vi "Day 03 (Part One).vi"() -> ()   [LabVIEW 2021]
panel:
  out "result":i32
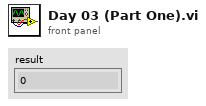
[diagram p1: front panel]
types:
  T1 = cluster{"number":i32, "start index":i32, "lenght":i32, "row":i32}
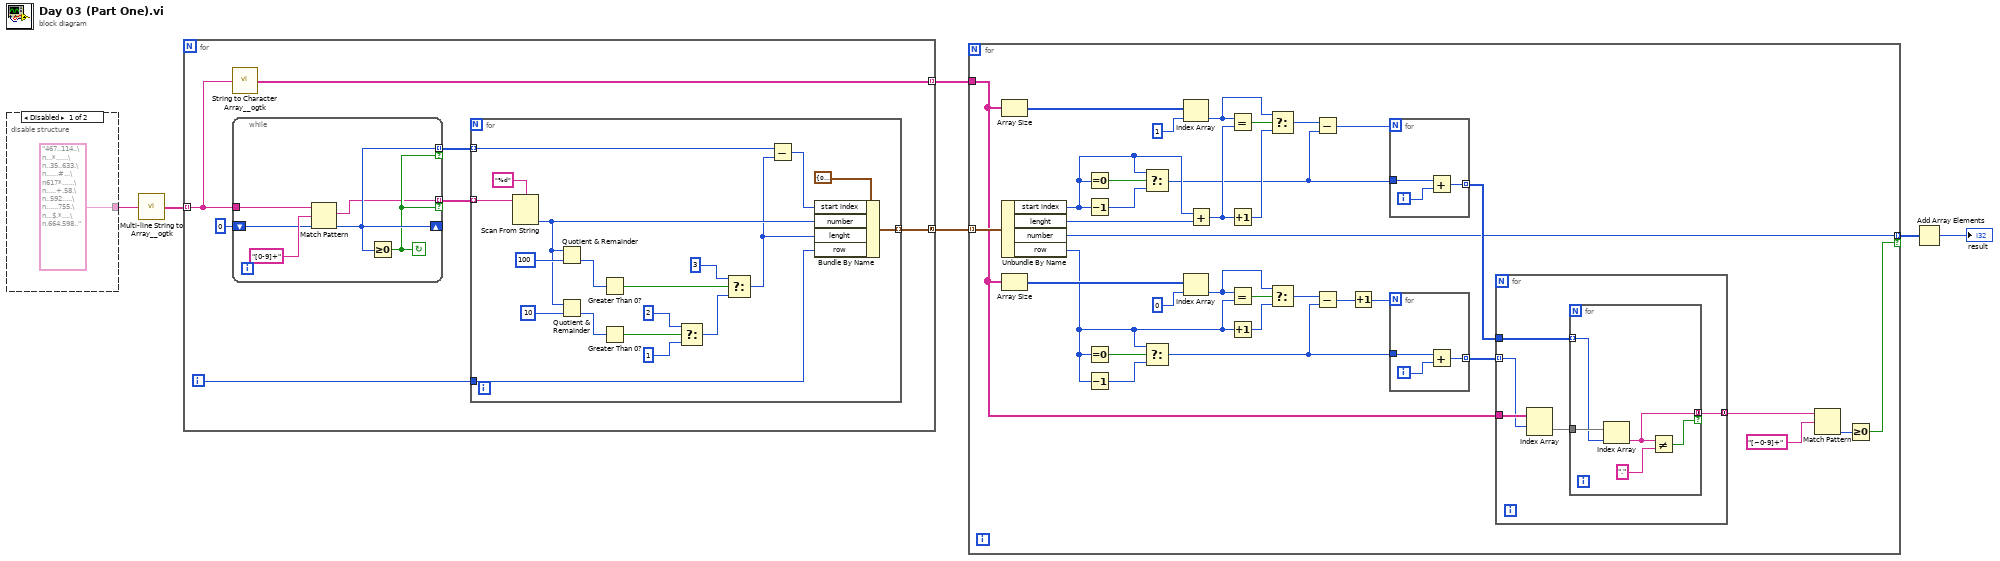
[diagram p0: block diagram]
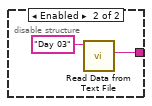
[diagram p2: hidden frame]
diagram:
  n1 = disable-structure shown="Disabled" {
    disable-tunnel: ["467..114..\n...*......\n..35..633.\n......#...\n617*......\n.....+.58.\n..592.....\n......755.\n...$.*....\n.664.598.." w9] -> w6
    frame Disabled {
    }
    frame Enabled {
      n2 = call "Read Data from Text File.vi"("Subfolder"="Day 03") -> ("data"=w9:string)  [unwired: 10 in]
    }
  }
  n3 = call <userlib>:"Multi-line String to Array__ogtk.vi"("string"=w6) -> ("lines"=w5:string[])
  n4 = for {
    tunnel: w5 -> [w12] mode=indexing
    tunnel: [w10] -> w4 mode=concatenating
    tunnel: [w11] -> w3 mode=indexing
    i -> [w13]
    n5 = call <userlib>:"String to Character Array__ogtk.vi"("Input String"=w12) -> ("Character Array"=w11:string[])
    n6 = while {
      tunnel: w12 -> [w41]
      shift-right: [w38] -> _
      shift-left: 0 ("offset past match") -> [w39]
      tunnel: [w36] -> w14 mode=indexing if=w37
      tunnel: [w38] -> w15 mode=indexing if=w37
      stop <- w37 continue-if-true
      n7 = Match Pattern(string=w41, regular expression="[0-9]+", offset (0)=w39) -> (match substring=w36:string, offset past match=w38:i32)  [unwired: 2 out]
      n8 = Greater Or Equal To 0?(x=w38) -> (x >= 0?=w37:bool)
    }
    n9 = for {
      tunnel: w15 -> [w19] mode=indexing
      tunnel: w14 -> [w34] mode=indexing
      tunnel: w13 -> [w32]
      tunnel: [w24] -> w10 mode=indexing
      n10 = Scan From String(format string="%d", input string=w34) -> (output 1=w23:i32)  [unwired: 3 in, 3 out]
      n11 = Quotient & Remainder(x=w23, y=100) -> (floor(x/y)=w25:i32)  [unwired: 1 out]
      n12 = Quotient & Remainder(x=w23, y=10) -> (floor(x/y)=w27:i32)  [unwired: 1 out]
      n13 = Greater Than 0?(x=w25) -> (x > 0?=w29:bool)
      n14 = Greater Than 0?(x=w27) -> (x > 0?=w28:bool)
      n15 = Select(t=2, s=w28, f=1) -> (s? t:f=w26:i32)
      n16 = Select(t=3, s=w29, f=w26) -> (s? t:f=w18:i32)
      n17 = Subtract(x=w19, y=w18) -> (x-y=w17:i32)
      n18 = Bundle By Name(cluster=T1 {"number"=0, "start index"=0, "lenght"=0, "row"=0}, "start index"=w17, "number"=w23, "lenght"=w18, "row"=w32) -> (w24:T1)
    }
  }
  n19 = for {
    tunnel: w4 -> [w75] mode=indexing
    tunnel: w3 -> [w48]
    tunnel: [w43] -> w2 mode=indexing if=w42
    n20 = Array Size(array=w48) -> (size(s)=w72:i32[])
    n21 = Unbundle By Name(w75) -> ("start index"=w69:i32, "lenght"=w70:i32, "number"=w43:i32, "row"=w58:i32)
    n22 = Array Size(array=w48) -> (size(s)=w61:i32[])
    n23 = Equal To 0?(x=w69) -> (x = 0?=w74:bool)
    n24 = Decrement(x=w69) -> (x-1=w73:i32)
    n25 = Equal To 0?(x=w58) -> (x = 0?=w59:bool)
    n26 = Decrement(x=w58) -> (x-1=w60:i32)
    n27 = Select(t=w69, s=w74, f=w73) -> (s? t:f=w51:i32)
    n28 = Select(t=w58, s=w59, f=w60) -> (s? t:f=w50:i32)
    n29 = Index Array(array=w72, index=1) -> (element=w67:i32)
    n30 = Index Array(array=w61, index=0) -> (element=w64:i32)
    n31 = Add(x=w69, y=w70) -> (x+y=w66:i32)
    n32 = Equal?(x=w67, y=w66) -> (x = y?=w68:bool)
    n33 = Increment(x=w66) -> (x+1=w55:i32)
    n34 = Equal?(x=w64, y=w58) -> (x = y?=w63:bool)
    n35 = Increment(x=w58) -> (x+1=w65:i32)
    n36 = Select(t=w67, s=w68, f=w55) -> (s? t:f=w57:i32)
    n37 = Select(t=w64, s=w63, f=w65) -> (s? t:f=w52:i32)
    n38 = Subtract(x=w57, y=w51) -> (x-y=w56:i32)
    n39 = Subtract(x=w52, y=w50) -> (x-y=w53:i32)
    n40 = Increment(x=w53) -> (x+1=w54:i32)
    n41 = for {
      N: w56 -> [_]
      tunnel: w51 -> [w91]
      tunnel: [w89] -> w47 mode=indexing
      i -> [w90]
      n42 = Add(x=w91, y=w90) -> (x+y=w89:i32)
    }
    n43 = for {
      N: w54 -> [_]
      tunnel: w50 -> [w88]
      tunnel: [w86] -> w49 mode=indexing
      i -> [w87]
      n44 = Add(x=w88, y=w87) -> (x+y=w86:i32)
    }
    n45 = for {
      tunnel: w49 -> [w78] mode=indexing
      tunnel: w48 -> [w79]
      tunnel: w47 -> [w80]
      tunnel: [w76] -> w46 mode=concatenating
      n46 = Index Array(array=w79, index (row)=w78) -> (element=w77:string[])  [unwired: 1 in]
      n47 = for {
        tunnel: w80 -> [w84] mode=indexing
        tunnel: w77 -> [w85]
        tunnel: [w83] -> w76 mode=concatenating if=w81
        n48 = Index Array(array=w85, index=w84) -> (element=w83:string)
        n49 = Not Equal?(x=w83, y=".") -> (x != y?=w81:bool)
      }
    }
    n50 = Match Pattern(string=w46, regular expression="[~0-9]+") -> (offset past match=w44:i32)  [unwired: 1 in, 3 out]
    n51 = Greater Or Equal To 0?(x=w44) -> (x >= 0?=w42:bool)
  }
  n52 = Add Array Elements(numeric array=w2) -> (sum=→"result":i32)
